vi "Mode 3 - AUT NF Characterization.vi"() -> (2 "Mode3 Test Properties":T1, 3 "Cancelled?":bool)   [LabVIEW 2018]
doc: "Use this template to create a dialog box with event handling."
uses:
  Mode3TestProperties.ctl
  Classes/Sequence/SequenceSubvis/RF Direction.ctl
panel:
  in  "VNA Calibration File":path
  in  "Data File Name":string
  in  "Probe Vertical Polarization":bool
  in  "Probe Horizontal Polarization":bool
  in  "Antenna Tx/Rx":bool
  in  "Upload TR Module file":path=path "C:/Users/Public/Documents/OU PAARD/mmWave_RF_Scanner/SupportFiles/Mode3example1.csv"
  in  "Cancel":bool
  in  "OK":bool
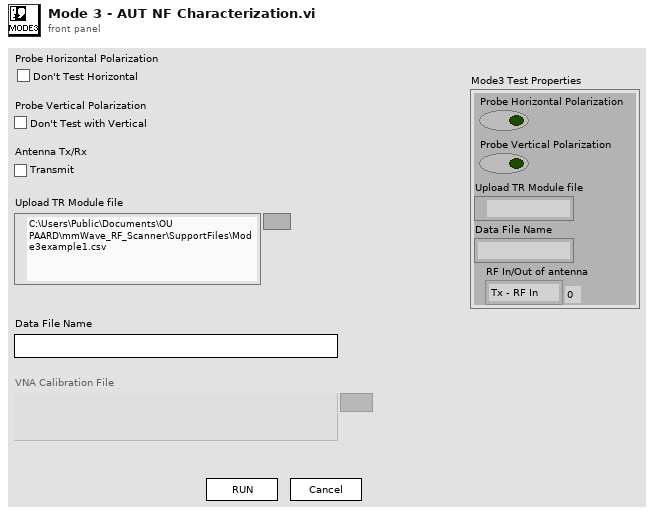
[diagram p1: front panel]
types:
  T1 = typedef "Mode3TestProperties.ctl" = cluster{"Probe Horizontal Polarization":bool, "Probe Vertical Polarization":bool, "Upload TR Module file":path, "Data File Name":string, "RF In/Out of antenna":T2}
  T2 = typedef "RF Direction.ctl" = enum16{"Tx - RF In", "Rx - RF Out"}
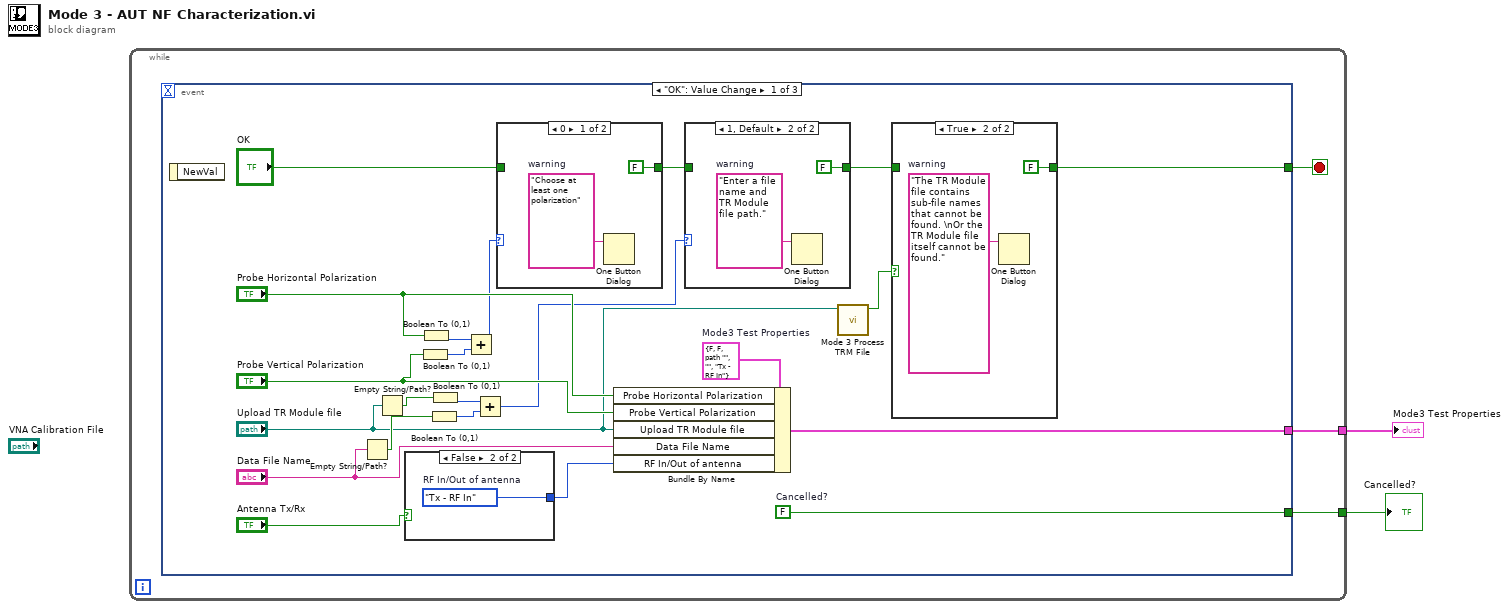
[diagram p0: block diagram]
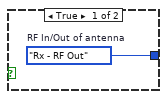
[diagram p5: hidden frame]
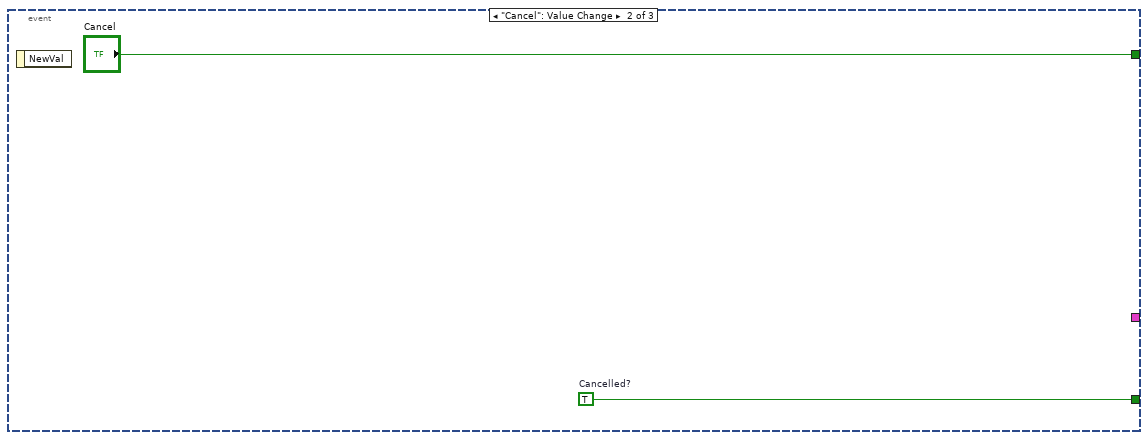
[diagram p6: hidden frame]
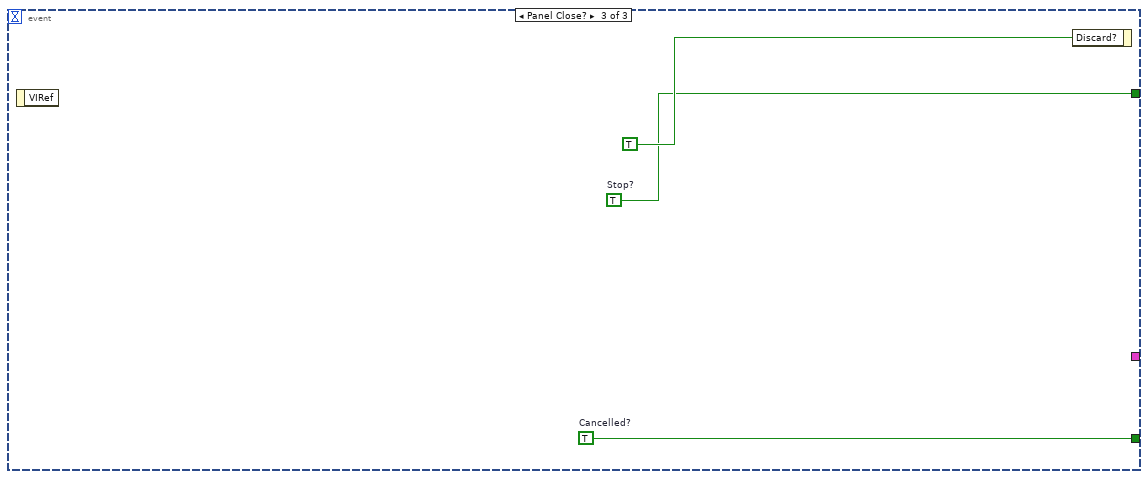
[diagram p7: hidden frame]
diagram:
  n1 = while {
    tunnel: [w4] -> w2
    tunnel: [w3] -> w1
    stop <- w5 stop-if-true
    n2 = event shown="[0] \"OK\": Value Change" {
      selector: _ -> [_ _ _]
      dyn-events: _ -> [_ _ _]
      timeout: _ -> [_ _ _]
      tunnel: [w6 "Cancel" w42] -> w5
      tunnel: [w27 w40 w41] -> w4
      tunnel: [w24 _ _] -> w3
      event "OK": Value Change {
        w10 = T1 {"Probe Horizontal Polarization"=FALSE, "Probe Vertical Polarization"=FALSE, "Upload TR Module file"=path "", "Data File Name"="", "RF In/Out of antenna"=enum."Tx - RF In"}  # Mode3 Test Properties
        w27 = FALSE  # Cancelled?
        n3 = event-data() -> ()  [unwired: 1 in, 1 out]
        n4 = Empty String/Path?(string/path="Data File Name") -> (empty?=w13:bool)
        n5 = Empty String/Path?(string/path="Upload TR Module file") -> (empty?=w14:bool)
        n6 = case shown="False" "Antenna Tx/Rx" {
          tunnel: [w37 w38] -> w25
          frame True {
            w37 = RF_Direction."Rx - RF Out"  # RF In/Out of antenna
          }
          frame False {
            w38 = RF_Direction."Tx - RF In"  # RF In/Out of antenna
          }
        }
        n7 = Boolean To (0,1)(Boolean="Probe Vertical Polarization") -> (0, 1=w22:i16)
        n8 = Boolean To (0,1)(Boolean="Probe Horizontal Polarization") -> (0, 1=w23:i16)
        n9 = Boolean To (0,1)(Boolean=w13) -> (0, 1=w16:i16)
        n10 = Boolean To (0,1)(Boolean=w14) -> (0, 1=w15:i16)
        n11 = Add(x=w23, y=w22) -> (x+y=w18:i16)
        n12 = Add(x=w15, y=w16) -> (x+y=w12:i16)
        n13 = case shown="0" w18 {
          tunnel: [FALSE w36] -> w11
          tunnel: "OK" -> [_ w36]
          frame 0 {
            w35 = "Choose at least one polarization"  # warning
            n14 = One Button Dialog(message=w35) -> ()  [unwired: 1 in, 1 out]
          }
          frame 1, Default {
          }
        }
        n15 = Bundle By Name(cluster=w10, "Probe Horizontal Polarization"="Probe Horizontal Polarization", "Probe Vertical Polarization"="Probe Vertical Polarization", "Upload TR Module file"="Upload TR Module file", "Data File Name"="Data File Name", "RF In/Out of antenna"=w25) -> (w24:T1)
        n16 = case shown="1, Default" w12 {
          tunnel: [w31 FALSE] -> w7
          tunnel: w11 -> [w31 _]
          frame 0 {
          }
          frame 1, Default {
            w33 = "Enter a file name and TR Module file path."  # warning
            n17 = One Button Dialog(message=w33) -> ()  [unwired: 1 in, 1 out]
          }
        }
        n18 = call "Mode 3 Process TRM File.vi"("Upload TR Module file"="Upload TR Module file") -> ("No file = True"=w8:bool)  [unwired: 8 in, 2 out]
        n19 = case shown="True" w8 {
          tunnel: [w28 FALSE] -> w6
          tunnel: w7 -> [w28 _]
          frame False {
          }
          frame True {
            w30 = "The TR Module file contains sub-file names that cannot be found. \nOr the TR Module file itself cannot be found."  # warning
            n20 = One Button Dialog(message=w30) -> ()  [unwired: 1 in, 1 out]
          }
        }
      }
      event "Cancel": Value Change {
        w40 = TRUE  # Cancelled?
        n21 = event-data() -> ()  [unwired: 1 in, 1 out]
      }
      event Panel Close? {
        w41 = TRUE  # Cancelled?
        w42 = TRUE  # Stop?
        n22 = event-data() -> ()  [unwired: 1 in, 1 out]
        n23 = event-data("Discard?"=TRUE) -> ()  [unwired: 1 in, 1 out]
      }
    }
  }
  "Cancelled?" <- w2
  "Mode3 Test Properties" <- w1
